vi "zmq_recv_timeout.vi"(4 "error in":errorcluster, 5 "timeout (ms)":u32=500, 7 "socket in":refnum<class "zmq_socket.lvclass">) -> (0 "error out":errorcluster, 1 "timeout?":bool, 2 "parts":string[](array[string]), 3 "socket out":refnum<class "zmq_socket.lvclass">)   [LabVIEW 2010, in "zeromq.lvlib" / "zmq_socket.lvclass"]
doc: "An implementation of \"receive with timeout\" functionality, returning an array of strings as per zmq_recv_multi. This VI is provided as a development \"crutch\" and is against the ZeroMQ philosophy but is highly convenient in some situations.\n\nPolls <b>socket in</b> periodically every <b>poll interval</b> milliseconds until a message has been received, or <b>timeout</b> milliseconds elapses since the start of the call. Aborts on error.\n\nDetailed API documentation: http://api.zeromq.org/3-2:zmq-poll"
uses:
  zmq_socket.lvclass
  zmq_socket.lvclass/zmq_socket.ctl
  <vilib>/Utility/error.llb/Error Cluster From Error Code.vi
  zeromq.lvlib
panel:
  # "ØMQ"
  # "labview"
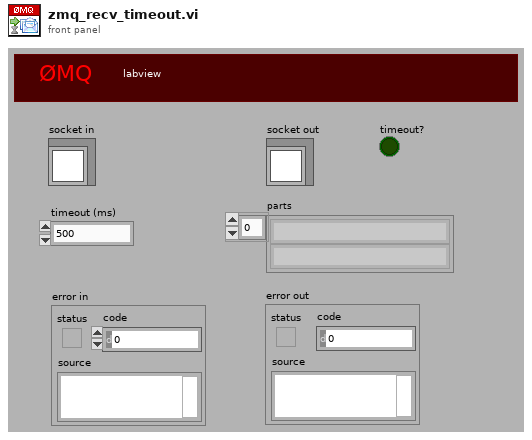
[diagram p1: front panel]
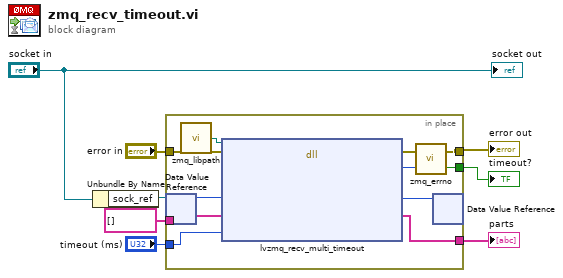
[diagram p0: block diagram]
diagram:
  n1 = Unbundle By Name("socket in") -> ("sock_ref"=w1:refnum<data-value>)
  n2 = in-place {
    in-place-border: string[] [] ("parts") -> [w19]
    in-place-border: [w18] -> w7
    in-place-border: "timeout (ms)" -> [w17]
    in-place-border: "error in" -> [w16]
    in-place-border: [w13] -> w4
    in-place-border: [w12] -> w3
    n3 = in-place-dvr #1(w1) -> (w11:u64)  [unwired: 1 out]
    n4 = call "zmq_libpath.vi"() -> ("path"=w9:path)
    n5 = dll-call lib="?" fn="lvzmq_recv_multi_timeout" ("zmq_labview.dll:lvzmq_socket")(path in=w9, error in=w16, "sock_obj"=w11, "data"=w19, "timeout"=w17) -> (error out=w15:errorcluster, "return type"=w14:i32, "sock_obj"=w10:u64, "data"=w18:string[])  [unwired: 4 in, 1 out]
    n6 = call "zmq_errno.vi"("retval"=w14, "error in"=w15) -> ("again?"=w12:bool, "error out"=w13:errorcluster)
    n7 = in-place-dvr #1(w10) -> ()  [unwired: 2 out]
  }
  "error out" <- w4
  "parts" <- w7
  "timeout?" <- w3
  "socket out" <- "socket in"
